vi "Create Differential Plot.vi"(6 "Upper Limit":dbl, 8 "Error In":errorcluster, 9 "Lower Limit":dbl, 10 "Dev2 Ch3":dynamicdata(waveform), 11 "Dev1 Ch3":dynamicdata(waveform)) -> (0 "Error Out":errorcluster, 3 "Array":cluster{"Array":dbl[], "Array":dbl[]}[](array[cluster]))   [LabVIEW 2017]
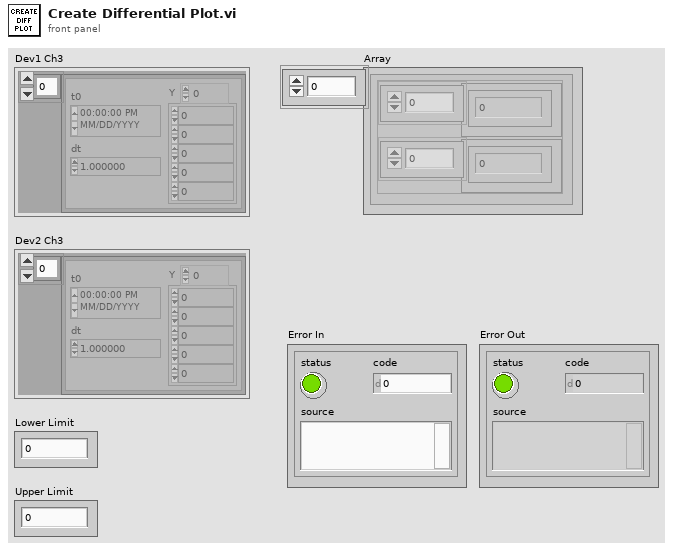
[diagram p1: front panel]
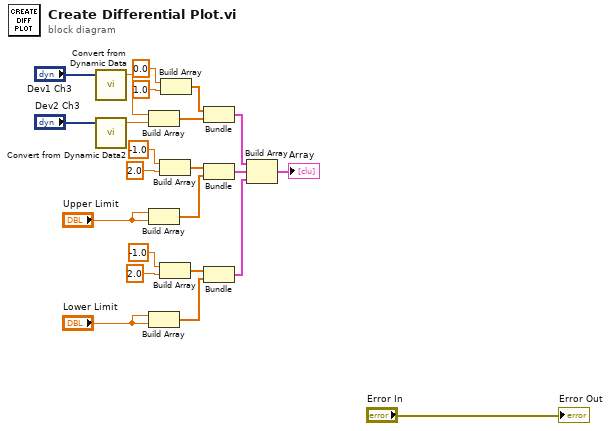
[diagram p0: block diagram]
diagram:
  n1 = call "Convert from Dynamic Data"("Dynamic Data Type"="Dev1 Ch3") -> ("Scalar"=w4:dbl)  [unwired: 3 in]
  n2 = call "Convert from Dynamic Data2"("Dynamic Data Type"="Dev2 Ch3") -> ("Scalar"=w7:dbl)  [unwired: 3 in]
  n3 = Build Array(w4, w7) -> (w8:dbl[])
  n4 = Build Array("Upper Limit", "Upper Limit") -> (w17:dbl[])
  n5 = Build Array("Lower Limit", "Lower Limit") -> (w19:dbl[])
  n6 = Build Array(-1.0 ("element"), 2.0 ("element")) -> (w15:dbl[])
  n7 = Build Array(-1.0 ("element"), 2.0 ("element")) -> (w18:dbl[])
  n8 = Build Array(0.0 ("element"), 1.0 ("element")) -> (w9:dbl[])
  n9 = Bundle(w9, w8) -> (w12:cluster{dbl[], dbl[]})  [unwired: 1 in]
  n10 = Bundle(w15, w17) -> (w13:cluster{dbl[], dbl[]})  [unwired: 1 in]
  n11 = Bundle(w18, w19) -> (w23:cluster{dbl[], dbl[]})  [unwired: 1 in]
  n12 = Build Array(w12, w13, w23) -> (→"Array":cluster{dbl[], dbl[]}[])
  "Error Out" <- "Error In"
